vi "Control Paths in Memory.vi"(4 "App":refnum<vi>) -> (7 "Control Paths":path[](array[path]))   [LabVIEW 2020, in "VolatusGUIEditor.lvlib"]
uses:
  VolatusGUIEditor.lvlib
  VolatusGUIEditorCore/VolatusControlsList/VolatusControlsList.lvclass
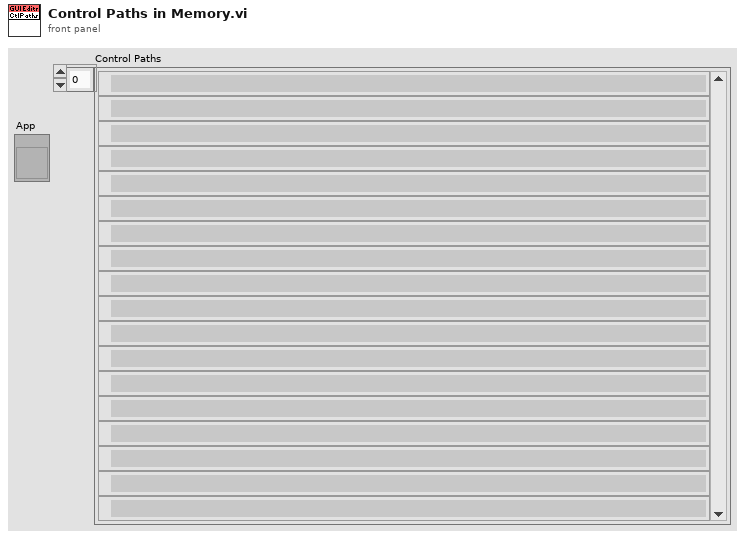
[diagram p1: front panel]
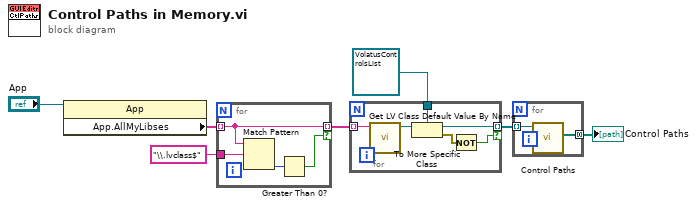
[diagram p0: block diagram]
diagram:
  n1 = property class="App"(reference="App") -> ("App.AllMyLibses"=w7:string[])  [unwired: 1 in, 2 out]
  n2 = for {
    tunnel: w7 -> [w10] mode=indexing
    tunnel: "\\.lvclass$" -> [w11]
    tunnel: [w10] -> w5 mode=indexing if=w8
    n3 = Match Pattern(string=w10, regular expression=w11) -> (offset past match=w9:i32)  [unwired: 1 in, 3 out]
    n4 = Greater Than 0?(x=w9) -> (x > 0?=w8:bool)
  }
  n5 = for {
    tunnel: w5 -> [w17] mode=indexing
    tunnel: refnum<class "VolatusControlsList.lvclass"> refnum ("VolatusGUIControls.lvlib:VolatusControlsList.lvclass") -> [w15]
    tunnel: [w14] -> w3 mode=indexing if=w12
    n6 = call <vilib>:"Get LV Class Default Value By Name.vi"("class name"=w17) -> ("object"=w16:refnum<class>)  [unwired: 9 in, 1 out]
    n7 = To More Specific Class(target class=w15, reference=w16) -> (specific class reference=w14:refnum<class "VolatusControlsList.lvclass">, error out=w13:errorcluster)  [unwired: 1 in]
    n8 = Not(x=w13) -> (.not. x?=w12:bool)
  }
  n9 = for {
    tunnel: w3 -> [w19] mode=indexing
    tunnel: [w18] -> w2 mode=concatenating
    n10 = call-dynamic "Control Paths.vi"("VolatusControlsList in"=w19) -> ("Control Paths"=w18:path[])  [unwired: 10 in]
  }
  "Control Paths" <- w2
